vi "transmit.vi"(8 "error in (no error)":errorcluster, 10 "RESP3 Value":variant, 11 "Redis TCP Client in":refnum<class "Redis TCP Client.lvclass">) -> (0 "error out":errorcluster, 3 "Redis TCP Client out":refnum<class "Redis TCP Client.lvclass">)   [LabVIEW 2019, in "Redis Client for LabVIEW.lvlib" / "Redis TCP Client.lvclass"]
uses:
  Redis TCP Client.lvclass
  Redis TCP Client.lvclass/Redis TCP Client.ctl
  lib/RESP3-for-LabVIEW/RESP3/RESP3.lvlib
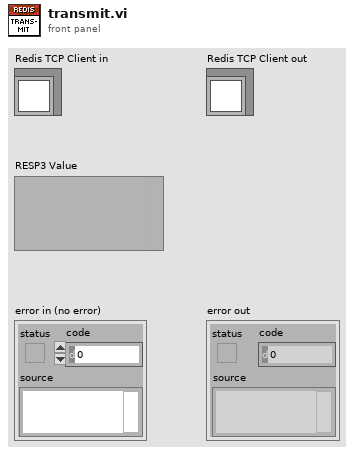
[diagram p1: front panel]
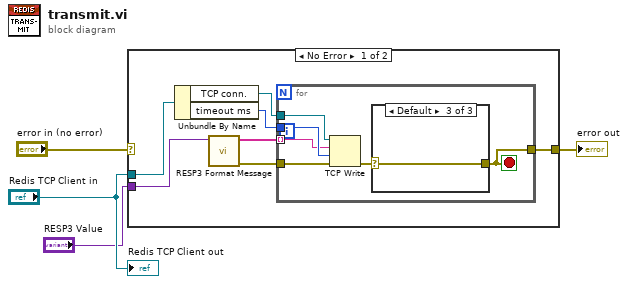
[diagram p0: block diagram]
diagram:
  n1 = case shown="No Error" "error in (no error)" {
    selector: "error in (no error)" -> [_ w19]
    tunnel: "Redis TCP Client in" -> [w11 _]
    tunnel: [w9 w19] -> w3
    tunnel: "RESP3 Value" -> [w7 _]
    frame No Error {
      n2 = Unbundle By Name(w11) -> ("TCP conn."=w8:refnum<k5>, "timeout ms"=w10:i32)
      n3 = call "RESP3 Format Message.vi"("RESP3 Value"=w7) -> ("error out"=w5:errorcluster, "messages"=w6:string[])  [unwired: 9 in]
      n4 = for {
        tunnel: w10 -> [w17]
        tunnel: [w13] -> w9
        tunnel: w8 -> [w15]
        tunnel: w6 -> [w14] mode=indexing
        tunnel: w5 -> [w12]
        stop <- w13 stop-if-true
        n5 = TCP Write(connection ID=w15, data in=w14, error in (no error)=w12, 9:w17) -> (error out=w16:errorcluster)  [unwired: 2 out]
        n6 = case shown="Default" w16 {
          selector: w16 -> [_ _ w18]
          tunnel: [_ _ w18] -> w13
          frame No Error {
          }
          frame Error {
          }
          frame Default {
          }
        }
      }
    }
    frame Error {
    }
  }
  "error out" <- w3
  "Redis TCP Client out" <- "Redis TCP Client in"
